vi "Make XML Param.vi"(8 "error in (no error)":errorcluster, 10 "Value":string, 11 "Name":string) -> (0 "error out":errorcluster, 3 "param":string)   [LabVIEW 2020, in "XmlInterface.lvclass"]
uses:
  XmlInterface.lvclass
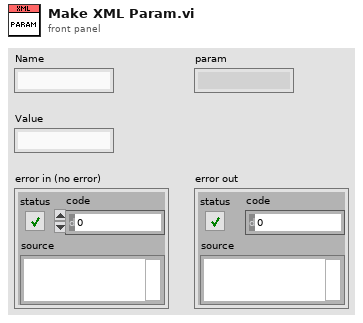
[diagram p1: front panel]
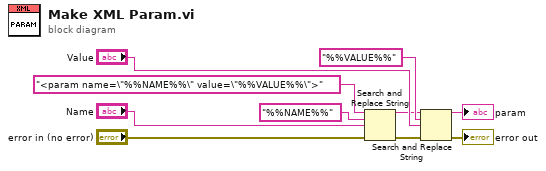
[diagram p0: block diagram]
diagram:
  n1 = Search and Replace String(input string="<param name=\"%%NAME%%\" value=\"%%VALUE%%\">", search string="%%NAME%%", replace string="Name", error in="error in (no error)") -> (result string=w6:string, error out=w4:errorcluster)  [unwired: 4 in, 2 out]
  n2 = Search and Replace String(input string=w6, search string="%%VALUE%%", replace string="Value", error in=w4) -> (result string=→"param":string, error out=→"error out":errorcluster)  [unwired: 4 in, 2 out]
